vi "Global FINE AVVIO.vi"() -> ()   [LabVIEW 2019]
panel:
  out "FINE FERMATA":bool
  out "AVVISO FERMATA IN CORSO":bool
  in  "vARM NOM DC":dbl
  out "STOP AFE ALTERNATORI":bool
  out "START AFE ALTERNATORI":bool
  out "Banco manuale":bool
  out "AVVISO AVVIO IN CORSO":bool
  out "FINE AVVIO":bool
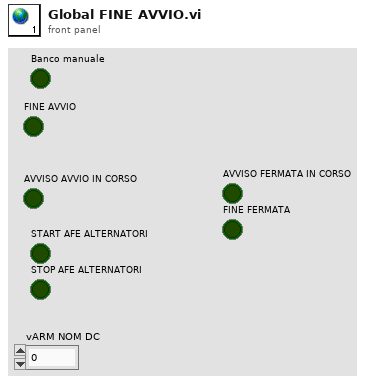
[diagram p1: front panel]
diagram:
